vi "convert_pixel_to_switch.vi"(11 "Pixel":u16) -> (3 "Switch":u16)   [LabVIEW 2016]
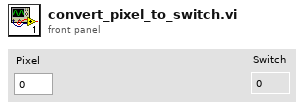
[diagram p1: front panel]
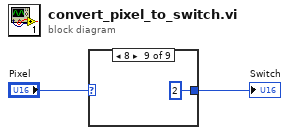
[diagram p0: block diagram]
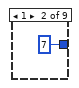
[diagram p3: hidden frame]
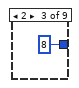
[diagram p4: hidden frame]
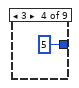
[diagram p5: hidden frame]
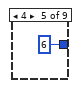
[diagram p6: hidden frame]
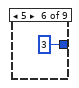
[diagram p7: hidden frame]
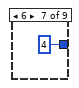
[diagram p8: hidden frame]
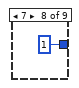
[diagram p9: hidden frame]
diagram:
  n1 = case shown="8" "Pixel" {
    selector: "Pixel" -> [w3 _ _ _ _ _ _ _ _]
    tunnel: [w3 u16 7 ("Numeric") u16 8 ("Numeric") u16 5 ("Numeric") u16 6 ("Numeric") u16 3 ("Numeric") u16 4 ("Numeric") u16 1 ("Numeric") u16 2 ("Numeric")] -> w1
    frame 0, Default {
    }
    frame 1 {
    }
    frame 2 {
    }
    frame 3 {
    }
    frame 4 {
    }
    frame 5 {
    }
    frame 6 {
    }
    frame 7 {
    }
    frame 8 {
    }
  }
  "Switch" <- w1
